vi "Typecast Refnum to Queue.vi"(11 "refnum in":T2) -> (3 "queue out":T1)   [LabVIEW 2017, in "DSF Configuration API.lvlib"]
uses:
  DSF Configuration API.lvlib
  Public/Controls/DSF Config Data RefNum.ctl
  Controls/Session/Config Queue.ctl
  Controls/Session/Config Data.ctl
  Controls/DSF File Format/DSF Config.ctl
  Public/Controls/Version Info.ctl
  Controls/DSF File Format/DSF Plugin.ctl
  Public/Controls/DSF Plugin Info.ctl
  Public/Controls/DSF Timing Info.ctl
  Controls/DSF File Format/DSF Group.ctl
  Public/Controls/DSF Group Info.ctl
  Controls/DSF File Format/DSF Transfer.ctl
  Public/Controls/DSF Transfer Info.ctl
  Controls/DSF File Format/DSF Channel.ctl
  Public/Controls/DSF Channel Info.ctl
  Controls/DSF File Format/DSF Settings.ctl
  Public/Controls/DSF Settings Info.ctl
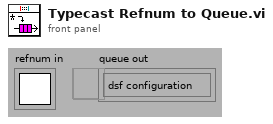
[diagram p1: front panel]
types:
  T1 = typedef "DSF Configuration API.lvlib/Config Queue.ctl" = refnum<queue>
  T2 = typedef "DSF Configuration API.lvlib/DSF Config Data RefNum.ctl" = refnum<k1>
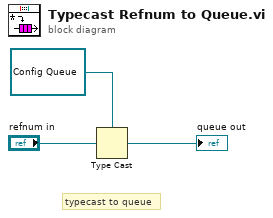
[diagram p0: block diagram]
diagram:
  # "typecast to queue"
  n1 = Type Cast(type=T1 refnum ("queue out"), x="refnum in") -> (*(type *) &x=→"queue out":T1)
